vi "Get Config.vi"(8 "error in (no error)":errorcluster) -> (0 "error out":errorcluster, 3 "Configur":T1)   [LabVIEW 2019, in "Full User Interface.lvlib"]
uses:
  Full User Interface.lvlib
  <vilib>/Test Bench Framework/Test Executive.lvlibp/TestEngine/TestEngine/TestEngine/Typedefs/TestEngine Cofiguration.ctl
  <vilib>/Test Bench Framework/Test Executive.lvlibp/TestEngine/TestEngine/TestEngine/Typedefs/Local Report Configuration.ctl
  <vilib>/Test Bench Framework/Test Executive.lvlibp/TestEngine/TestEngine/TestEngine/Report Format.ctl
  <vilib>/Test Bench Framework/Test Executive.lvlibp/TestEngine/TestEngine/TestEngine/Typedefs/Database Configuration.ctl
  <vilib>/Test Bench Framework/Test Executive.lvlibp/TestEngine/TestEngine/TestEngine/Test Engine.lvclass
  <vilib>/Utility/config.llb/NI_LVConfig.lvlib
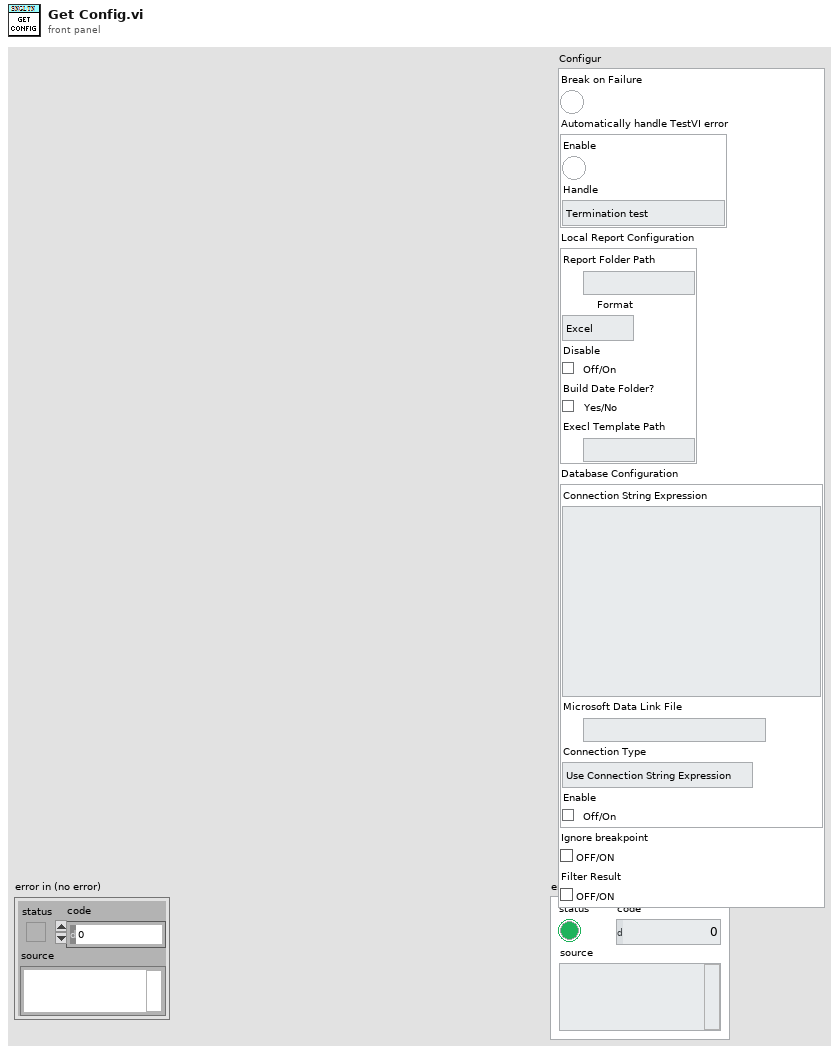
[diagram p1: front panel]
types:
  T1 = typedef "Test Executive.lvlibp/Test Engine.lvlib/Test Engine.lvclass/TestEngine Cofiguration.ctl" = cluster{"Break on Failure":bool, "Automatically handle TestVI error":cluster{"Enable":bool, "Handle":enum16{"Termination test", "Ignore error"}}, "Local Report Configuration":T2, "Database Configuration":T4, "Ignore breakpoint":bool, "Filter Result":bool}
  T2 = typedef "Test Executive.lvlibp/Test Engine.lvlib/Test Engine.lvclass/Local Report Configuration.ctl" = cluster{"Report Folder Path":path, "Format":T3, "Disable":bool, "Build Date Folder?":bool, "Execl Template Path":path}
  T3 = typedef "Test Executive.lvlibp/Test Engine.lvlib/Test Engine.lvclass/Report Format.ctl" = enum16{"Excel", "CSV(Tab)", "CSV(,)", "CSV(;)", "TEXT", "HTML"}
  T4 = typedef "Test Executive.lvlibp/Test Engine.lvlib/Test Engine.lvclass/Database Configuration.ctl" = cluster{"Connection String Expression":string, "Microsoft Data Link File":path, "Connection Type":enum16{"Use Connection String Expression", "Use Microsoft Data Link File"}, "Enable":bool}
  T5 = typedef "NI_LVConfig.lvlib/Config Data RefNum.ctl" = refnum<k1>
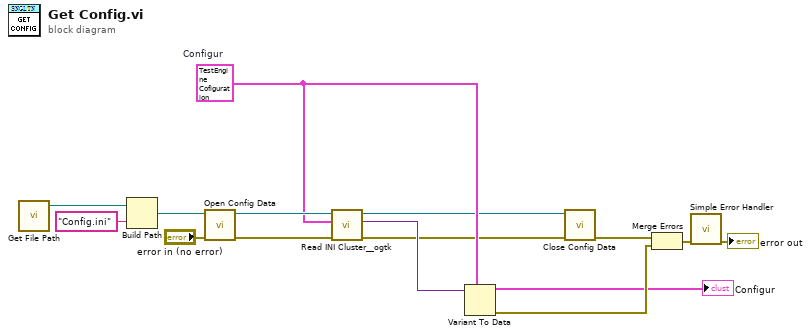
[diagram p0: block diagram]
diagram:
  w9 = T1 {"Break on Failure"=FALSE, "Automatically handle TestVI error"={"Enable"=FALSE, "Handle"=enum."Termination test"}, "Local Report Configuration"={"Report Folder Path"=path "", "Format"=enum."Excel", "Disable"=FALSE, "Build Date Folder?"=FALSE, "Execl Template Path"=path ""}, "Database Configuration"={"Connection String Expression"="", "Microsoft Data Link File"=path "", "Connection Type"=enum."Use Connection String Expression", "Enable"=FALSE}, "Ignore breakpoint"=FALSE, "Filter Result"=FALSE}  # Configur
  n1 = call "Get File Path.vi"() -> ("Application Directory"=w13:path)  [unwired: 11 in]
  n2 = Build Path(base path=w13, name or relative path="Config.ini") -> (appended path=w11:path)
  n3 = call <vilib>:"Open Config Data.vi"("error in (no error)"="error in (no error)", "configuration file path"=w11) -> ("error out"=w14:errorcluster, "refnum"=w15:T5)  [unwired: 7 in, 1 out]
  n4 = call <userlib>:"Read INI Cluster__ogtk.vi"("error in (no error)"=w14, "INI Fomatted Cluster Type"=w9, "refnum"=w15) -> ("error out"=w7:errorcluster, "INI Fomatted Cluster"=w10:variant, "dup refnum"=w8:T5)  [unwired: 4 in, 2 out]
  n5 = Variant To Data(type=w9, Variant=w10) -> (data=→"Configur":T1, error out=w4:errorcluster)  [unwired: 1 in]
  n6 = call <vilib>:"Close Config Data.vi"("error in (no error)"=w7, "refnum"=w8) -> ("error out"=w5:errorcluster)  [unwired: 8 in, 1 out]
  n7 = Merge Errors(w5, w4) -> (w3:errorcluster)
  n8 = call <vilib>:"Simple Error Handler.vi"("error in (no error)"=w3) -> ("error out"=→"error out":errorcluster)  [unwired: 4 in, 4 out]
